vi "getTY.vi"() -> ()   [LabVIEW 2019]
uses:
  <vilib>/Rock Robotics/Network Tables/NT Write Number.vi
  <vilib>/Rock Robotics/Network Tables/NT Read Number.vi
panel:
  in  "Numeric":dbl=1.0 format="%#_13g"
  in  "Numeric 3":dbl=1.0 format="%#_13g"
  in  "Name":string="Numeric"
  out "d":dbl
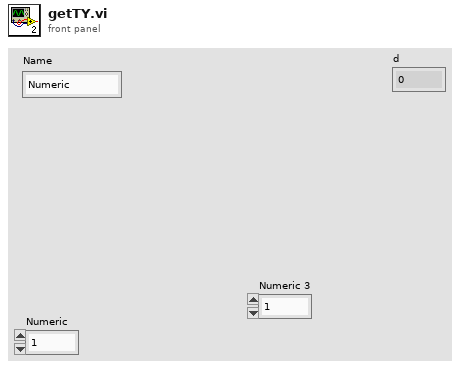
[diagram p1: front panel]
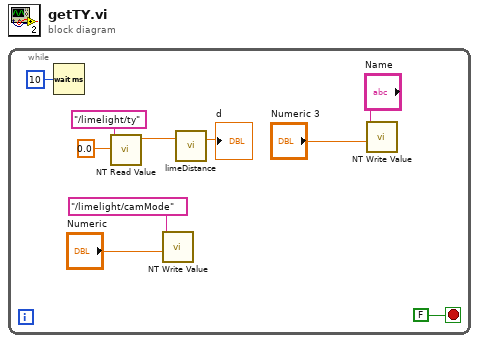
[diagram p0: block diagram]
diagram:
  n1 = while {
    stop <- FALSE stop-if-true
    n2 = Wait (ms)(milliseconds to wait=u32 10) -> ()  [unwired: 1 out]
    n3 = call-poly <vilib>:"NT Read Value.vi"("Default Value"=0.0 ("Numeric"), "Name"="/limelight/ty") -> ("Numeric"=w1:dbl)  [unwired: 8 in, 1 out]
    n4 = call-poly <vilib>:"NT Write Value.vi"("Numeric"="Numeric", "Name"="/limelight/camMode") -> ()  [unwired: 9 in, 1 out]
    n5 = call "limeDistance.vi"("a2"=w1) -> ("d"=→"d":dbl)  [unwired: 10 in]
    n6 = call-poly <vilib>:"NT Write Value.vi"("Numeric"="Numeric 3", "Name"="Name") -> ()  [unwired: 9 in, 1 out]
  }
